vi "RT.vi"() -> ()   [LabVIEW 2020]
uses:
  source/Client/Client/Client.lvclass
  source/Value/Value.lvlib
panel:
  in  "PV name":string
  out "Alarm":string
  out "Description":string
  out "Value":string
  out "Timestamp":timestamp
  out "timed out?":bool
  in  "Timeout":dbl[unit]=1.0
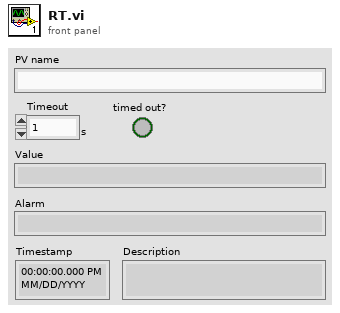
[diagram p1: front panel]
types:
  T1 = typedef "Value.lvlib/Display Metadata.ctl" = cluster{"Limit Low":dbl, "Limit High":dbl, "Description":string, "Units":string, "Precision":i32, "Form":enum32{"Default", "String", "Binary", "Decimal", "Hex", "Exponential", "Engineering"}}
  T2 = typedef "Value.lvlib/Alarm Severity.ctl" = enum32{"no", "minor", "major", "record", "invalid", "undefined", ""}
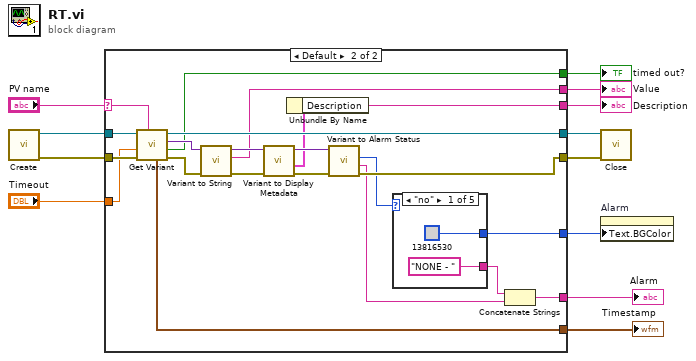
[diagram p0: block diagram]
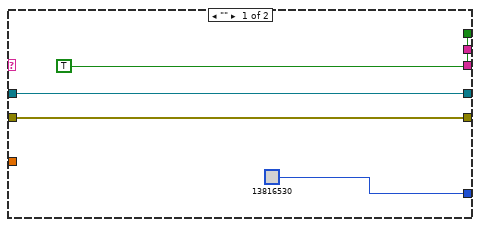
[diagram p2: hidden frame]
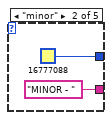
[diagram p3: hidden frame]
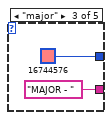
[diagram p4: hidden frame]
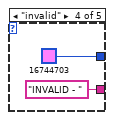
[diagram p5: hidden frame]
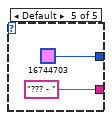
[diagram p6: hidden frame]
diagram:
  n1 = call "Create.vi"() -> ("error out"=w9:errorcluster, "Client out"=w10:refnum<class "Client.lvclass">)  [unwired: 10 in]
  n2 = case shown="Default" "PV name" {
    selector: "PV name" -> [_ w36]
    tunnel: w9 -> [w15 w38]
    tunnel: w10 -> [w16 w37]
    tunnel: [w16 w35] -> w12
    tunnel: [w15 w28] -> w11
    tunnel: [u32 13816530 ("Text.BGColor") w24] -> w7
    tunnel: [_ w23] -> w6
    tunnel: [_ w22] -> w5
    tunnel: [TRUE w21] -> w4
    tunnel: "Timeout" -> [_ w20]
    tunnel: [_ w19] -> w2
    tunnel: [_ w17] -> w1
    frame "" {
    }
    frame Default {
      n3 = call "Get Variant.vi"("PV name"=w36, "error in"=w38, "timeout"=w20, "Client in"=w37) -> ("error out"=w33:errorcluster, "timed out?"=w21:bool, "value"=w34:variant, "Client out"=w35:refnum<class "Client.lvclass">, "timestamp"=w19:timestamp)  [unwired: 3 in]
      n4 = call "Variant to String.vi"("error in"=w33, "value"=w34) -> ("error out"=w32:errorcluster, "string"=w22:string, "value dup"=w31:variant)  [unwired: 7 in]
      n5 = call "Variant to Display Metadata.vi"("error in"=w32, "value"=w31) -> ("error out"=w30:errorcluster, "display metadata"=w18:T1, "value out"=w29:variant)  [unwired: 6 in, 1 out]
      n6 = Unbundle By Name(w18) -> ("Description"=w17:string)
      n7 = call "Variant to Alarm Status.vi"("error in"=w30, "value"=w29) -> ("error out"=w28:errorcluster, "Message"=w25:string, "Severity"=w27:T2)  [unwired: 5 in, 2 out]
      n8 = case shown="\"no\"" w27 {
        tunnel: [u32 13816530 ("Text.BGColor") u32 16777088 ("Text.BGColor") u32 16744576 ("Text.BGColor") u32 16744703 ("Text.BGColor") u32 16744703 ("Text.BGColor")] -> w24
        tunnel: ["NONE - " "MINOR - " "MAJOR - " "INVALID - " "??? - "] -> w26
        frame "no" {
        }
        frame "minor" {
        }
        frame "major" {
        }
        frame "invalid" {
        }
        frame Default {
        }
      }
      n9 = Concatenate Strings(w26, w25) -> (w23:string)
    }
  }
  "Alarm" <- w6
  "Description" <- w1
  "Value" <- w5
  "Timestamp" <- w2
  "timed out?" <- w4
  n10 = call "Close.vi"("error in (no error)"=w11, "Client in"=w12) -> ()  [unwired: 9 in, 1 out]
  n11 = property on="Alarm" class="Str"("Text.BGColor"=w7) -> ()  [unwired: 2 in, 2 out]
